vi "pitch.vi"() -> ()   [LabVIEW 2009]
panel:
  out "pitch":dbl
  in  "q3":i16
  in  "q2":i16
  in  "q1":i16
  in  "q0":i16
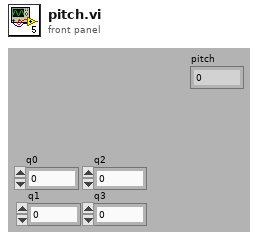
[diagram p1: front panel]
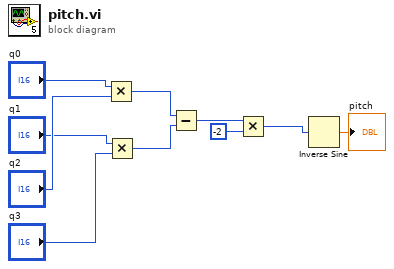
[diagram p0: block diagram]
diagram:
  n1 = Multiply(x="q0", y="q2") -> (x*y=w6:i16)
  n2 = Multiply(x="q1", y="q3") -> (x*y=w5:i16)
  n3 = Subtract(x=w6, y=w5) -> (x-y=w4:i16)
  n4 = Multiply(x=w4, y=i16 -2) -> (x*y=w2:i16)
  n5 = Inverse Sine(1:w2) -> (0:→"pitch":dbl)
